vi "Preview Vacuum State.vi"(8 "error in (no error)":errorcluster, 10 "timeout in ms (-1)":i32=-1, 11 "cRIO-CO2 in":refnum<class "cRIO-CO2.lvclass">) -> (0 "error out":errorcluster, 1 "State":T1, 2 "Pressure (mBar)":dbl, 3 "cRIO-CO2 out":refnum<class "cRIO-CO2.lvclass">, 4 "timed out?":bool, 5 "Vacuum StateQ":refnum<queue>, 6 "Raw Pressure":dbl)   [LabVIEW 2015, in "cRIO-Carbondioxide.lvlib" / "cRIO-CO2.lvlib" / "cRIO-CO2.lvclass"]
uses:
  cRIO-CO2.lvclass
  Controls/Vacuum State Cluster.ctl
  Controls/Vacuum State Enumerator.ctl
  cRIO-CO2.lvclass/cRIO-CO2.ctl
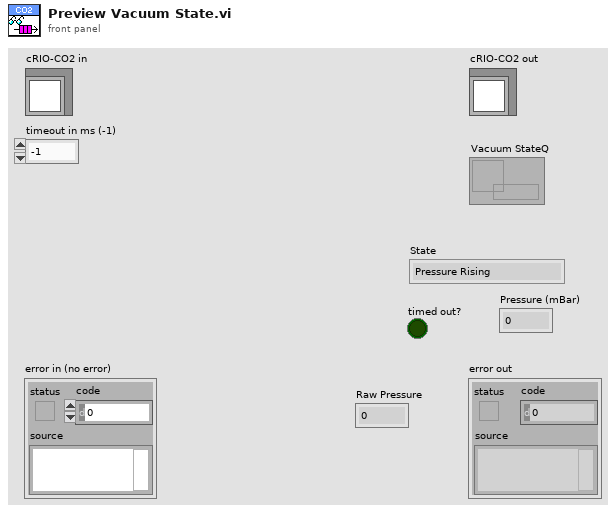
[diagram p1: front panel]
types:
  T1 = typedef "Vacuum State Enumerator.ctl" = enum16{"Pressure Rising", "Plateau", "Pressure Dropping", "Valley", "Low Valley", "Leak", "Unknown"}
  T2 = typedef "Vacuum State Cluster.ctl" = cluster{"Vacuum State":T1, "Pressure":dbl, "Raw Pressure":dbl, "d/dt":dbl}
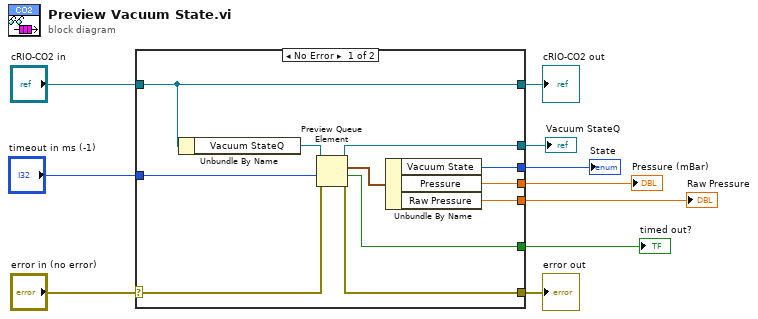
[diagram p0: block diagram]
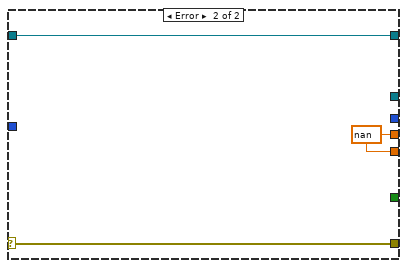
[diagram p2: hidden frame]
diagram:
  n1 = case shown="No Error" "error in (no error)" {
    selector: "error in (no error)" -> [w20 w23]
    tunnel: [w19 w23] -> w9
    tunnel: [w21 w24] -> w7
    tunnel: "cRIO-CO2 in" -> [w21 w24]
    tunnel: [w11 _] -> w6
    tunnel: "timeout in ms (-1)" -> [w17 _]
    tunnel: [w14 _] -> w4
    tunnel: [w15 _] -> w3
    tunnel: [w13 w22] -> w2
    tunnel: [w12 w22] -> w1
    frame No Error {
      n2 = Unbundle By Name(w21) -> ("Vacuum StateQ"=w18:refnum<queue>)
      n3 = Preview Queue Element(queue=w18, timeout in ms (-1)=w17, error in (no error)=w20) -> (queue out=w11:refnum<queue>, element=w16:T2, timed out?=w15:bool, error out=w19:errorcluster)
      n4 = Unbundle By Name(w16) -> ("Vacuum State"=w14:T1, "Pressure"=w13:dbl, "Raw Pressure"=w12:dbl)
    }
    frame Error {
      w22 = nan ("Pressure")
    }
  }
  "error out" <- w9
  "cRIO-CO2 out" <- w7
  "Vacuum StateQ" <- w6
  "State" <- w4
  "timed out?" <- w3
  "Pressure (mBar)" <- w2
  "Raw Pressure" <- w1
